vi "Process-error-caller.vi"(8 "error in (no error)":errorcluster, 11 "Errors in":T1) -> (0 "error out":errorcluster, 3 "Errors out":T1)   [LabVIEW 2013, in "Error-handling.lvlib" / "Errors.lvclass"]
uses:
  Errors.lvclass
  Object-reference.ctl
  Errors.lvclass/Errors.ctl
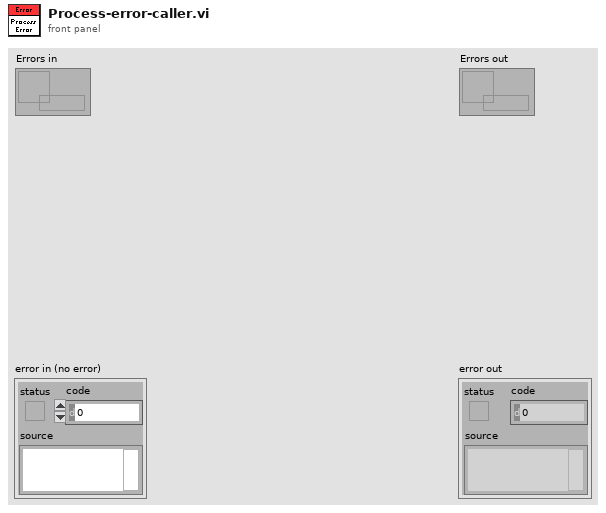
[diagram p1: front panel]
types:
  T1 = typedef "Error-handling.lvlib/Errors.lvclass/Object-reference.ctl" = refnum<data-value>
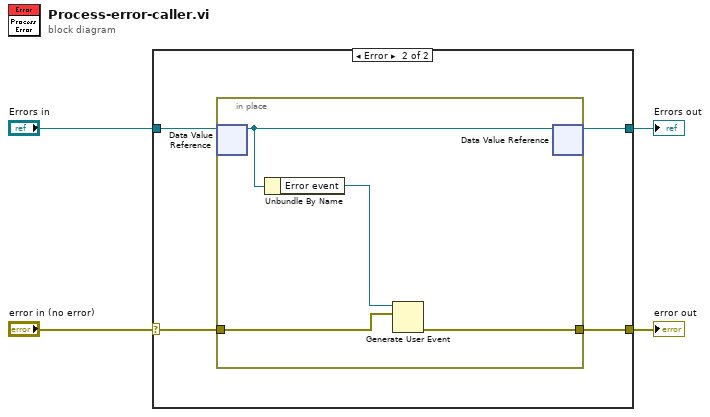
[diagram p0: block diagram]
diagram:
  n1 = case shown="Error" "error in (no error)" {
    selector: "error in (no error)" -> [w5 w8]
    tunnel: [w5 w7] -> w3
    tunnel: [w6 w9] -> w1
    tunnel: "Errors in" -> [w6 w10]
    frame No Error {
    }
    frame Error {
      n2 = in-place {
        in-place-border: w8 -> [w13]
        in-place-border: [w12] -> w7
        n3 = in-place-dvr #1(w10) -> (w11:refnum<class "Errors.lvclass">)  [unwired: 1 out]
        n4 = Unbundle By Name(w11) -> ("Error event"=w14:refnum<user-event>)
        n5 = Generate User Event(user event=w14, event data cluster=w13) -> (error out=w12:errorcluster)  [unwired: 2 in, 1 out]
        n6 = in-place-dvr #1(w11) -> (w9:T1)  [unwired: 1 out]
      }
    }
  }
  "error out" <- w3
  "Errors out" <- w1
